vi "MOVIE_close_movie_acquisition_sCMOS.vi"(2 "error in":errorcluster, 3 "parameters path":path, 4 "Global parameters":T1={"405"=0.0, "488"=0.0, "561"=0.0, "641"=0.0, "BF"=0.0, "X"=0.0, "Y"=0.0, "Filter list"=1, "Exp time"=0.0, "Kinetic time"=0.0, "Gain"=0, "Step length (nm)"=0, "Total range (nm)"=0, "Scan illumination\n mode"=FALSE, "Dt (s)"=0, "# repetitions"=0} {"# repetitions" min=0; "Dt (s)" min=0 step=1; "Filter list" items=["ET665lp", "zet405/488/561/640m", "None", "None", "None", "None"]}) -> (0 "error out":errorcluster)   [LabVIEW 2015]
uses:
  CONTROLS/Global parameters.ctl
panel:
  in  "Start acquisition":bool
  out "Global parameters I":T1 {"# repetitions" min=0; "Dt (s)" min=0 step=1; "Filter list" items=["ET665lp", "zet405/488/561/640m", "None", "None", "None", "None"]}
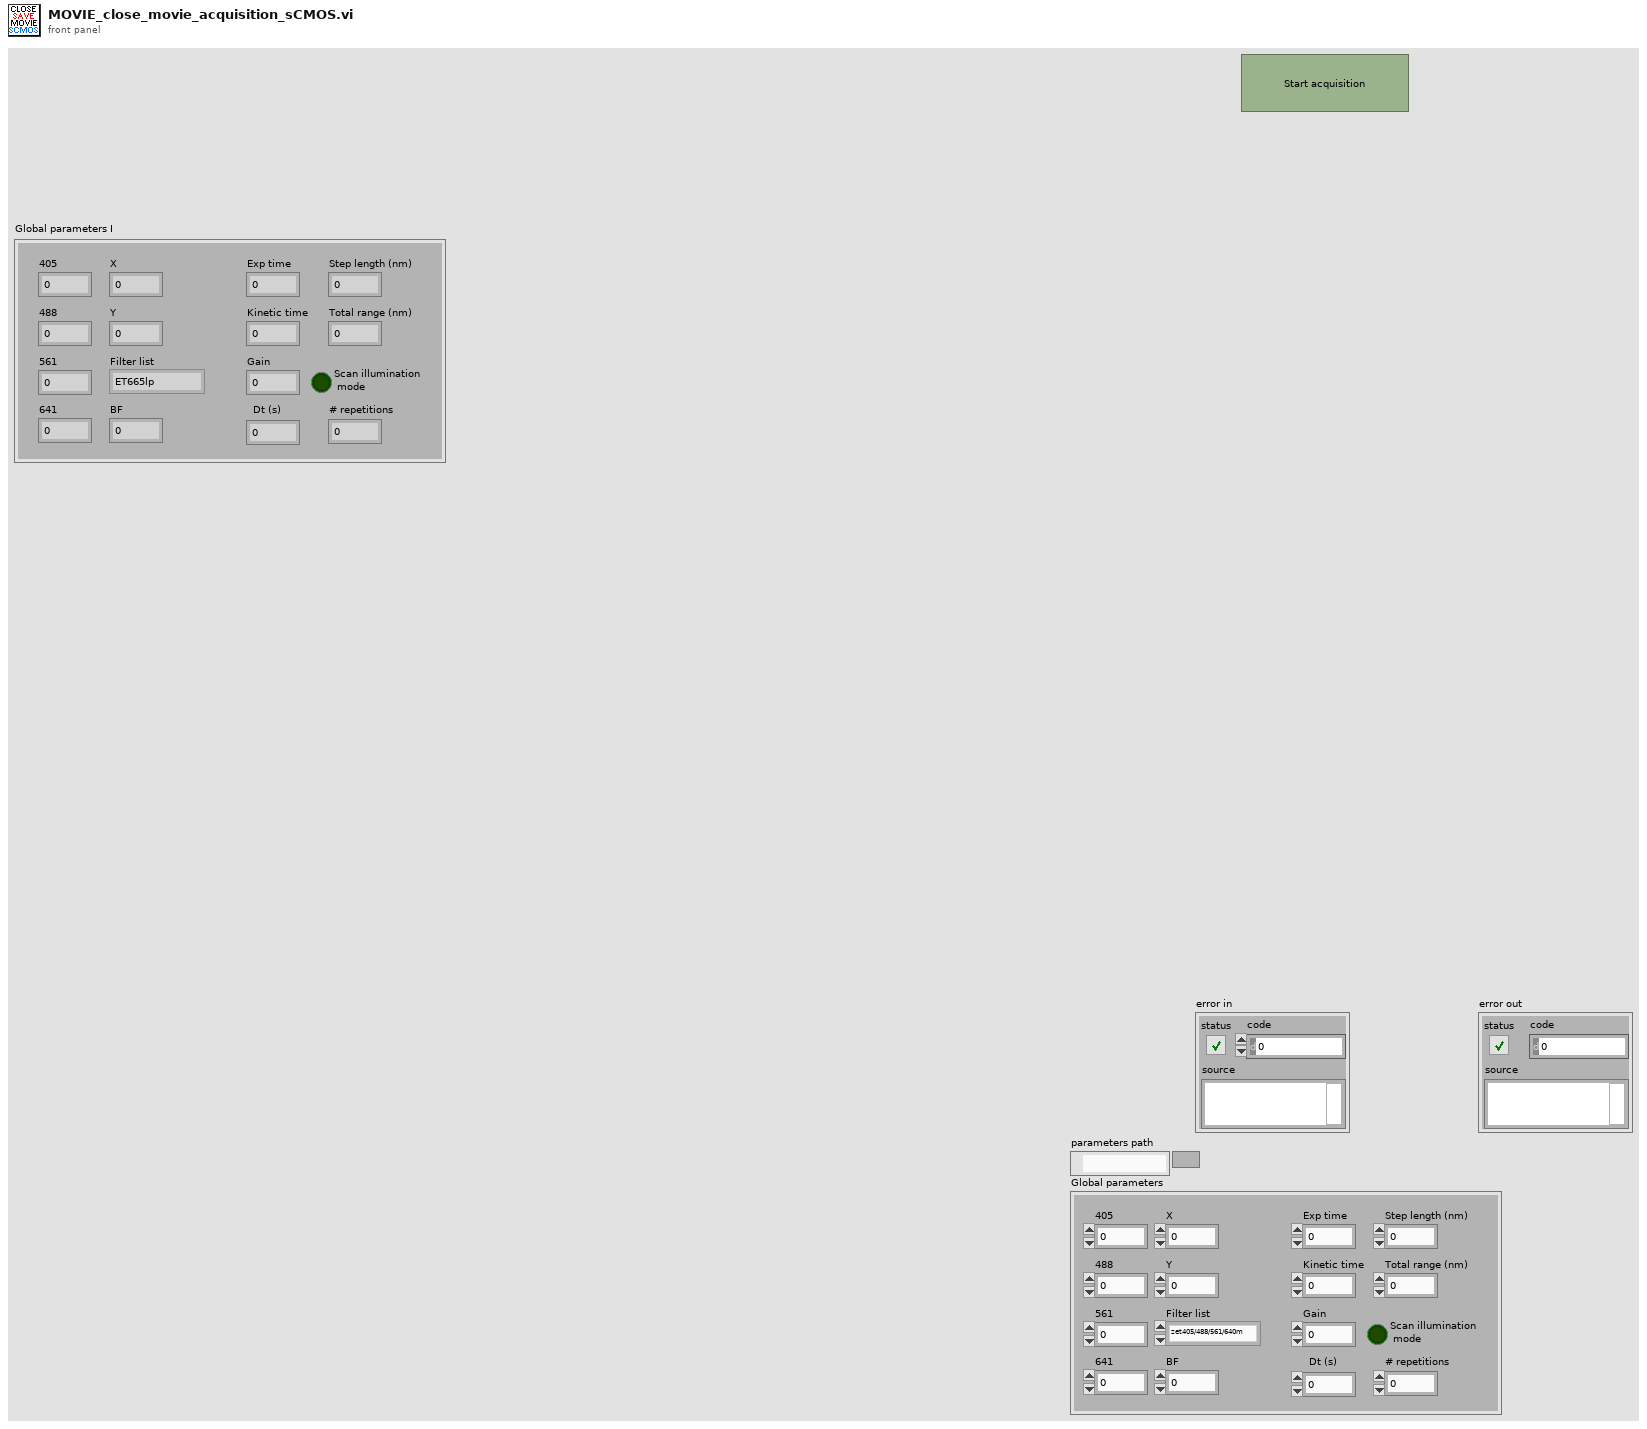
[diagram p1: front panel]
types:
  T1 = typedef "Global parameters.ctl" = cluster{"405":dbl, "488":dbl, "561":dbl, "641":dbl, "BF":dbl, "X":dbl, "Y":dbl, "Filter list":u16, "Exp time":sgl, "Kinetic time":sgl, "Gain":i32, "Step length (nm)":u32, "Total range (nm)":u32, "Scan illumination\n mode":bool, "Dt (s)":i32, "# repetitions":i32}
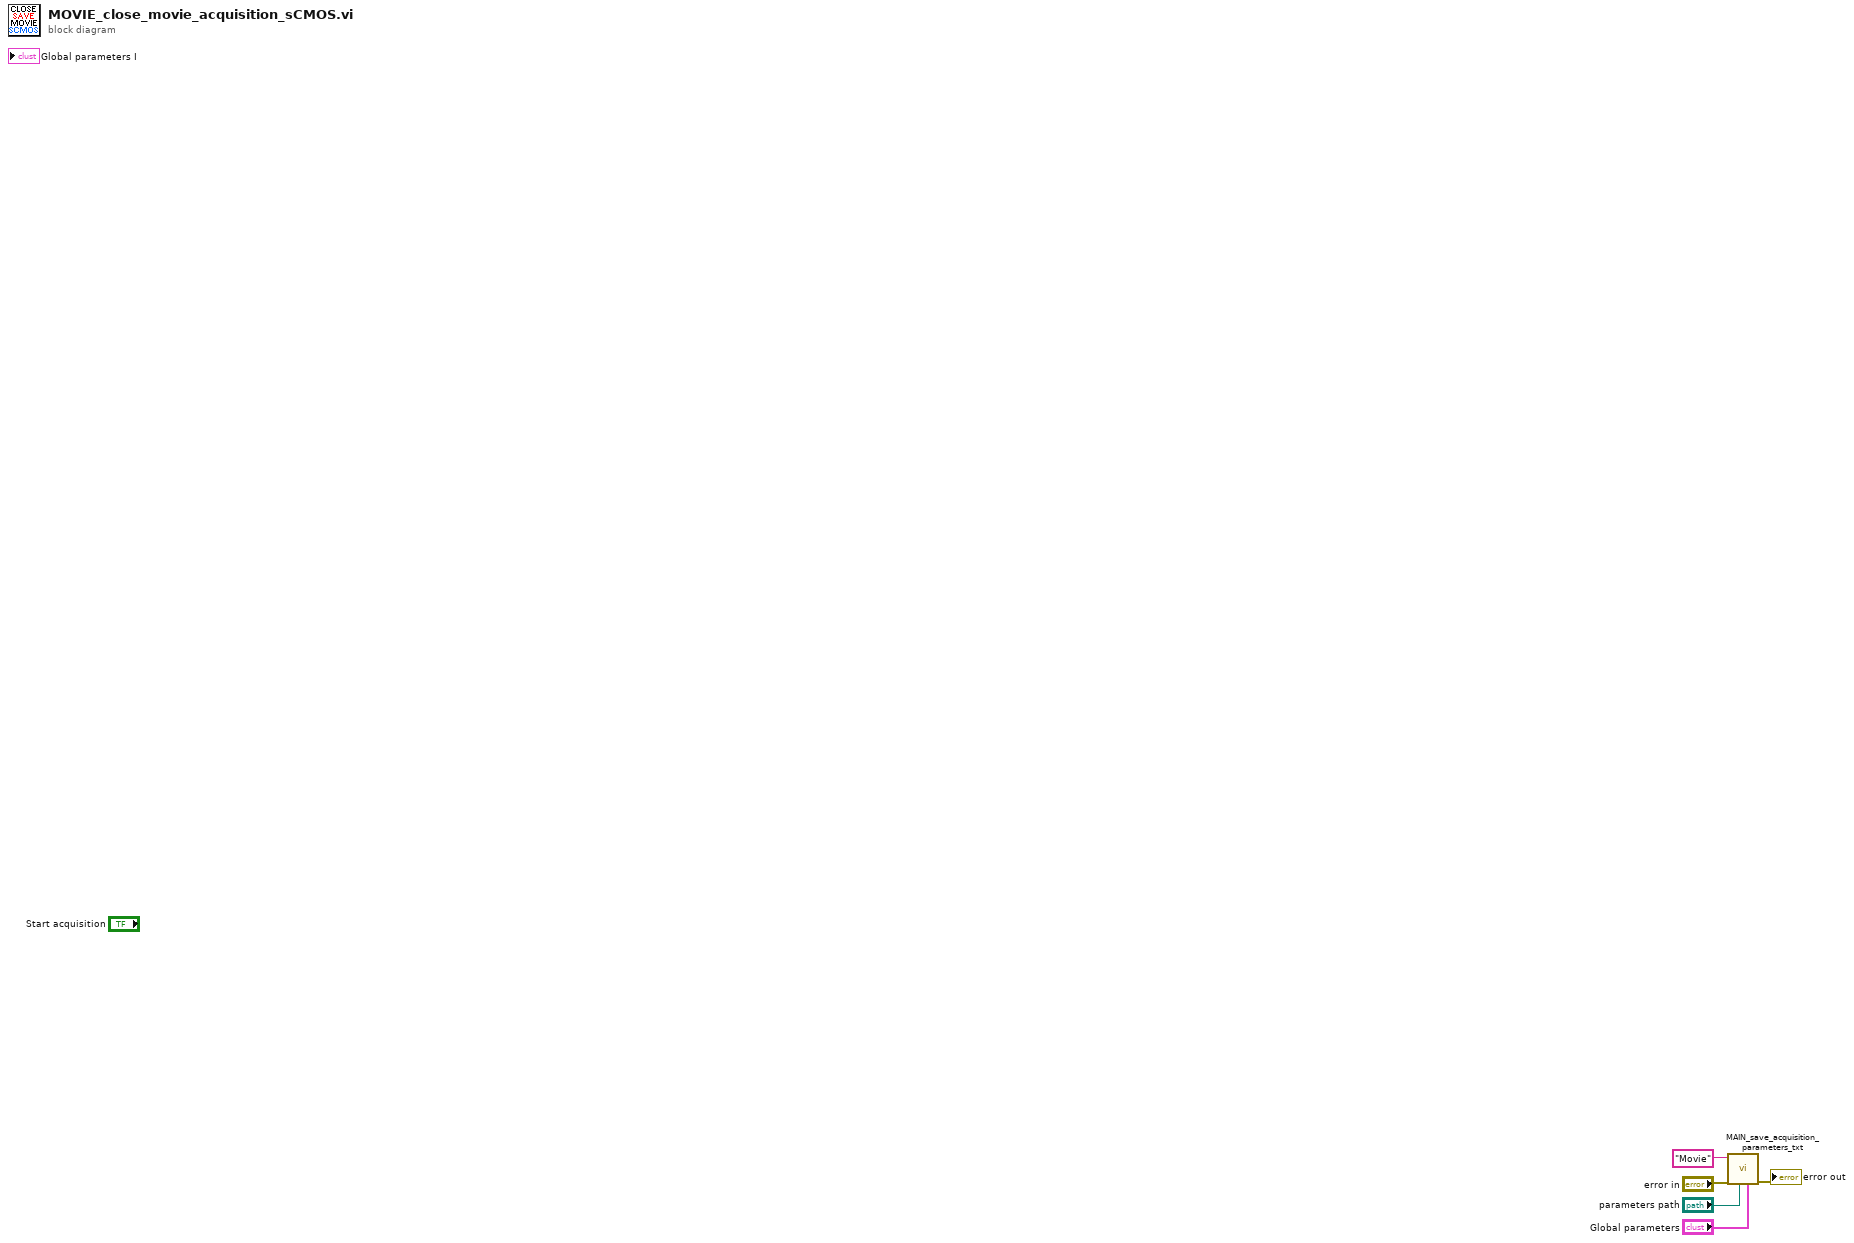
[diagram p0: block diagram]
diagram:
  n1 = call "MAIN_save_acquisition_parameters_txt.vi"("Global parameters"="Global parameters", "file path"="parameters path", "error in"="error in", "Data type"="Movie") -> ("error out"=→"error out":errorcluster)  [unwired: 7 in]
